vi "PIDAutoTune_ClosedLoopStep.vi"(7 "Configuration Parameters":T2={"Controller Constant Type"=enum."Ziegler Nicols - Normal", "Type of Controller"=enum."PI", "CO Offset"=0.25, "Kn"=1.0, "Tuning Tolerance"=0.001, "Plant Tolerance"=0.001, "Newest Avg Time "=1, "Long Ave Time"=6}, 8 "Sampling Time dt (s)":dbl=0.02, 9 "Tune":bool, 10 "Measurement  (PV)":dbl, 11 "Control Output (Co)":dbl) -> (0 "Plant and Test Data":T4, 1 "New Tuning Parameters":T3, 2 "Tuning Done":bool, 3 "Adj CO":dbl, 4 "Error Occured":bool, 6 "Diagnostic":T1)   [LabVIEW 2019, in "Trajectory_Library.lvlib"]
uses:
  Trajectory_Library.lvlib
  <vilib>/addons/control/pid/NI_PID_autopid.lvlib
  <vilib>/ptbypt/NI_PtbyPt.lvlib
  <vilib>/Analysis/Matrix/NI_Matrix.lvlib
  <vilib>/addons/control/pid/autopid.llb/PID Autotuning Design (Auto).vi
  <vilib>/addons/control/pid/autopid.llb/PID Autotuning Design (Chien-Hrones-Reswick).vi
  <vilib>/Analysis/Matrix/Numeric/Conversions/Array To Matrix - RA.vi
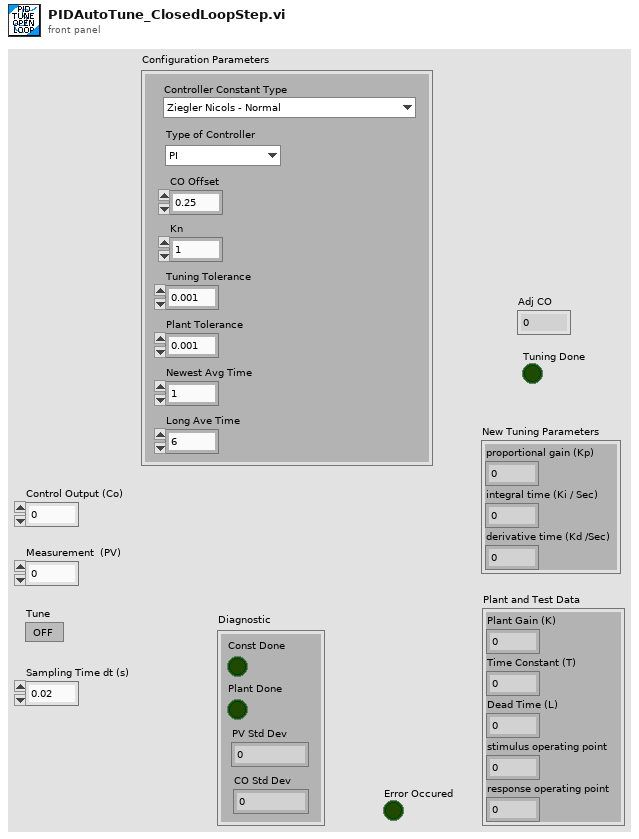
[diagram p1: front panel]
types:
  T1 = cluster{"Const Done":bool, "Plant Done":bool, "PV Std Dev":dbl, "CO Std Dev":dbl}
  T2 = cluster{"Controller Constant Type":enum16{"Ziegler Nicols - Fast", "Ziegler Nicols - Normal", "Ziegler Nicols - Slow", "CHR regulator - 0% overshoot", "CHR regulator - 20% overshoot", "CHR servo - 0 % overshoot", "CHR servo - 20% overshoot"}, "Type of Controller":enum16{"P", "PI", "PID"}, "CO Offset":dbl, "Kn":dbl, "Tuning Tolerance":dbl, "Plant Tolerance":dbl, "Newest Avg Time ":i32, "Long Ave Time":i32}
  T3 = cluster{"proportional gain (Kp)":dbl, "integral time (Ki / Sec)":dbl, "derivative time (Kd /Sec)":dbl}
  T4 = cluster{"Plant Gain (K)":dbl, "Time Constant (T)":dbl, "Dead Time (L)":dbl, "stimulus operating point":dbl, "response operating point":dbl}
  T5 = enum16{"Moving Average", "Low Pass 1st Order Butterworth", "Low Pass 2nd Order Butterworth", "High Pass 1st Order Butterworth", "High Pass 2nd Order Butterworth"}
  T6 = enum16{"Ziegler Nicols - Fast", "Ziegler Nicols - Normal", "Ziegler Nicols - Slow", "CHR regulator - 0% overshoot", "CHR regulator - 20% overshoot", "CHR servo - 0 % overshoot", "CHR servo - 20% overshoot"}
  T7 = cluster{"proportional gain (Kc)":dbl, "integral time (Ti, min)":dbl, "derivative time (Td, min)":dbl}
  T8 = cluster{"Plant Gain (K)":dbl, "Time Constant (T)":dbl, "Dead Time (L)":dbl}
  T9 = cluster{"Plant Gain (K)":dbl, "Time Constant (T)":dbl, "Dead Time (L)":dbl, "stimulus offset":dbl, "response offset":dbl}
  T10 = typedef "NI_Matrix.lvlib/RealMatrix.ctl" = dbl[][]
  T11 = cluster{"WithinTolerance":bool, "WithinTolerance":bool, "standard deviation":dbl, "standard deviation":dbl}
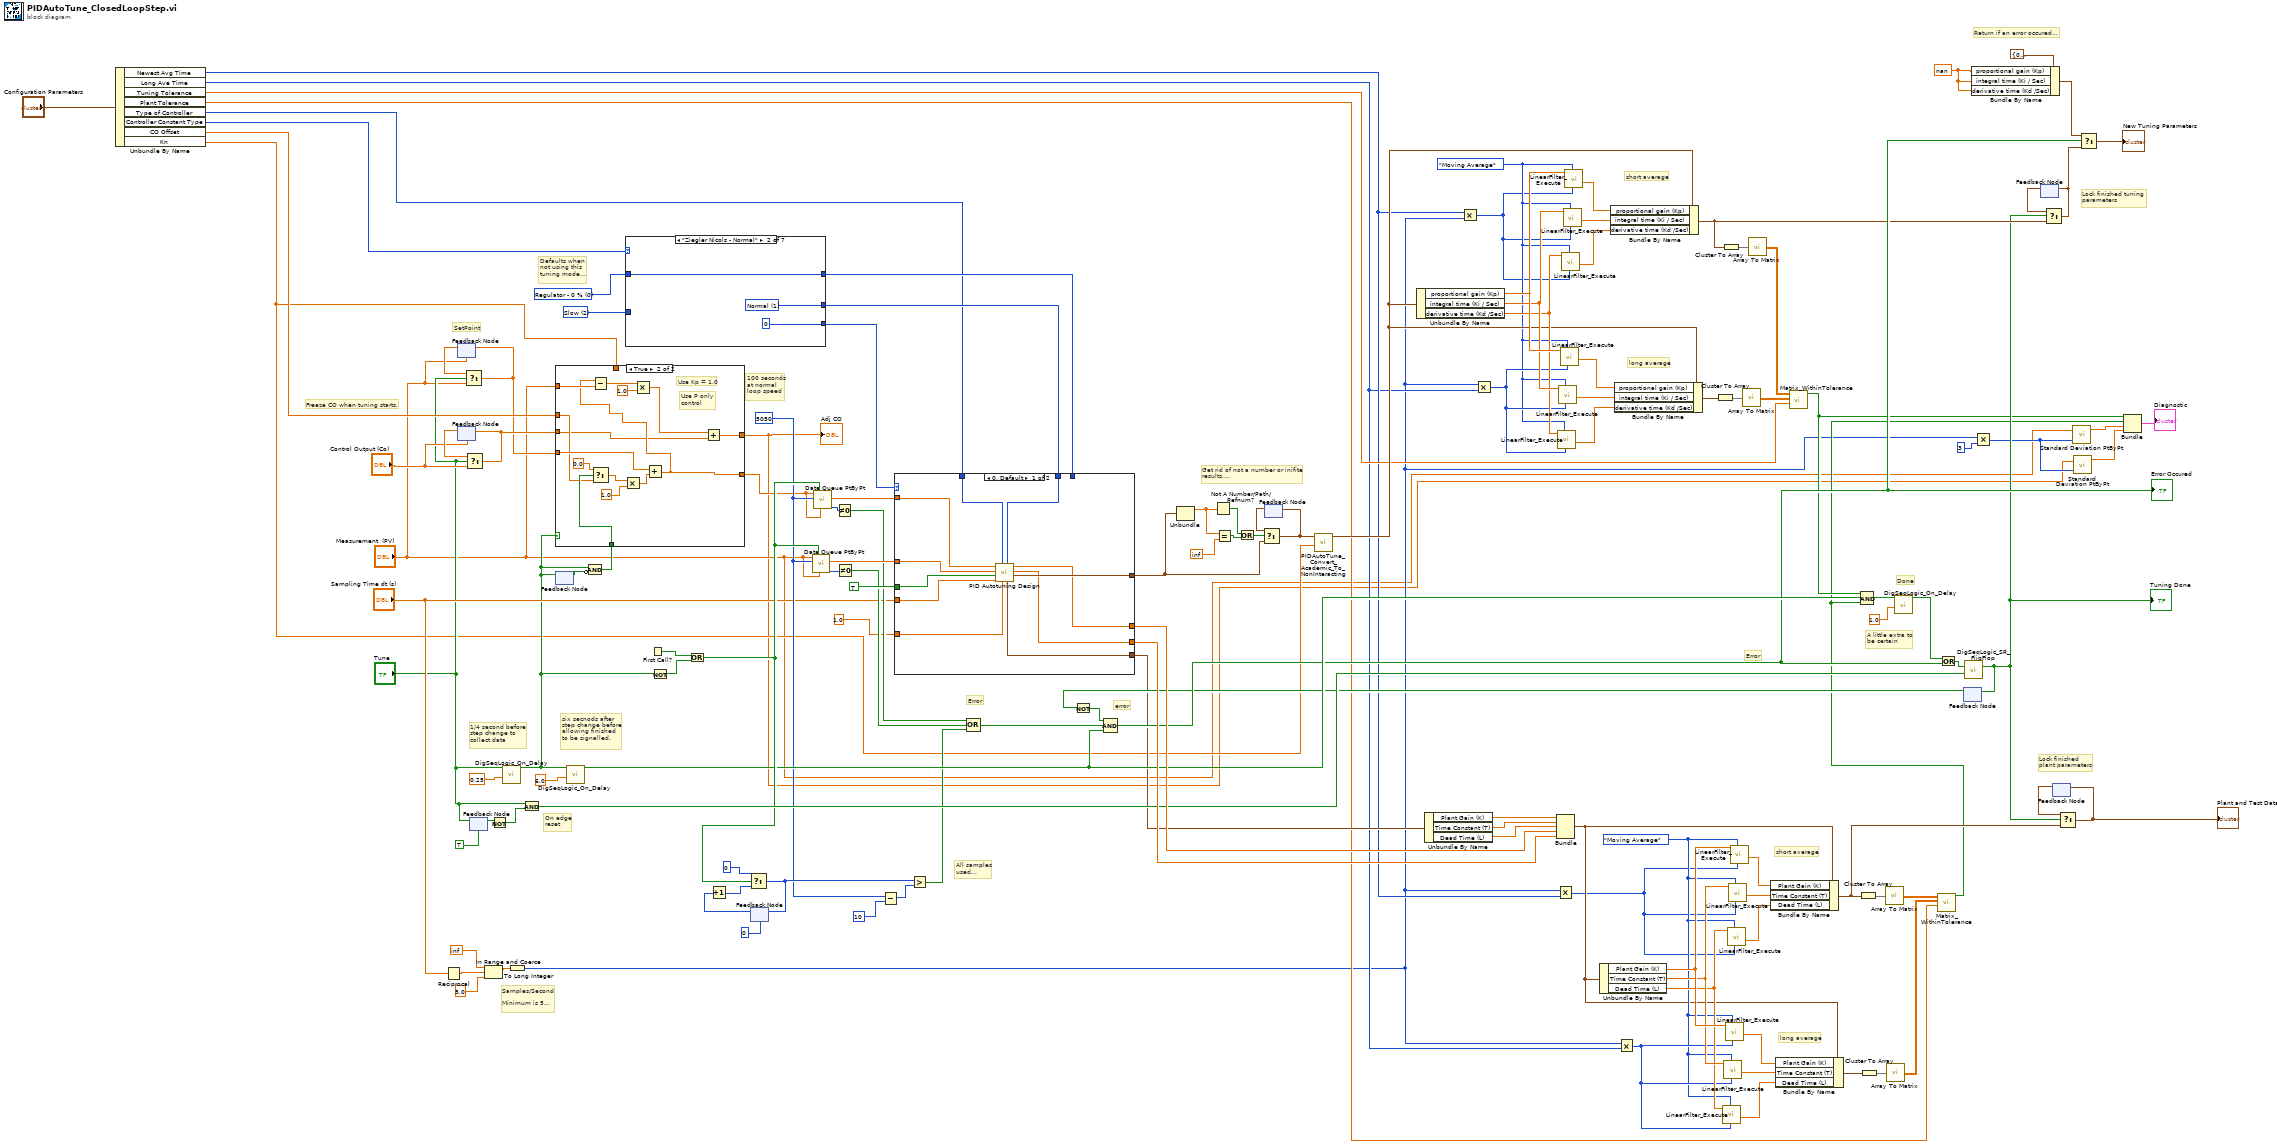
[diagram p0: block diagram]
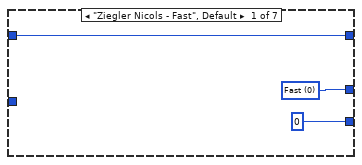
[diagram p2: hidden frame]
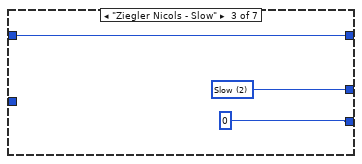
[diagram p3: hidden frame]
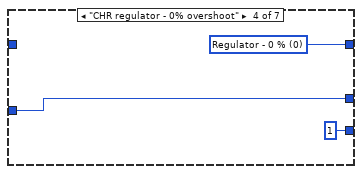
[diagram p4: hidden frame]
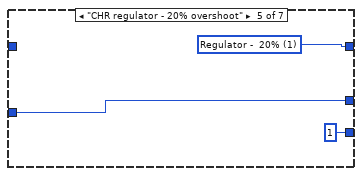
[diagram p5: hidden frame]
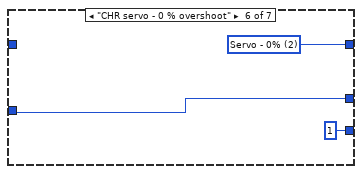
[diagram p6: hidden frame]
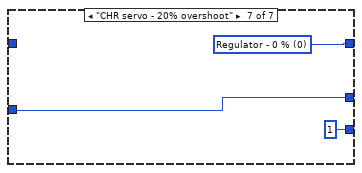
[diagram p7: hidden frame]
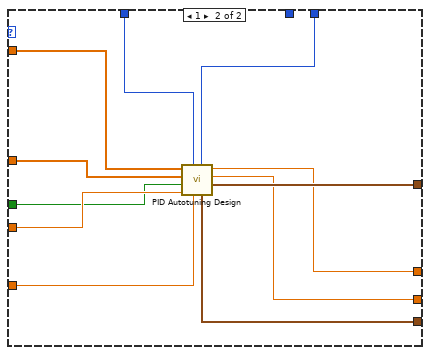
[diagram p8: hidden frame]
diagram:
  w39 = T5."Moving Average" ("Filter Type")
  w91 = nan
  w50 = T5."Moving Average" ("Filter Type")
  w106 = u16 2 items=["Fast", "Normal", "Slow"] ("Ziegler-Nichols Speed")
  w107 = u16 0 items=["Regulator - 0 %", "Regulator -  20%", "Servo - 0%", "Servo - 20%"] ("Tuning specifications")
  w78 = 5050 ("sample length")
  # "SetPoint"
  # "Get rid of not a number or inifite\nresults...."
  # "On edge\nreset"
  # "Error"
  # "All samples\nused..."
  # "Error"
  # "Done"
  # "Lock finished \nplant parameters"
  # "Lock finished tuning\nparameters"
  # "Samples/Second\n\nMinimum is 5..."
  # "long average"
  # "short average"
  # "long average"
  # "short average"
  # "error"
  # "Return if an error occured..."
  # "A little extra to\nbe certain"
  # "Defaults when\nnot using this\ntuning mode..."
  # "100 seconds\nat normal\nloop speed"
  # "Freeze CO when tuning starts."
  # "six secnods after\nstep change before\nallowing finished \nto be signalled."
  # "1/4 second before\nstep change to\ncollect data"
  n1 = Unbundle By Name("Configuration Parameters") -> ("Newest Avg Time"=w21:i32, "Long Ave Time"=w20:i32, "Tuning Tolerance"=w26:dbl, "Plant Tolerance"=w25:dbl, "Type of Controller"=w28:enum16{"P", "PI", "PID"}, "Controller Constant Type"=w29:T6, "CO Offset"=w27:dbl, "Kn"=w9:dbl)
  n2 = Reciprocal(x="Sampling Time dt (s)") -> (1/x=w68:dbl)
  n3 = feedback #1("Measurement  (PV)") -> (w16:dbl)
  n4 = feedback #2("Control Output (Co)") -> (w121:dbl)
  n5 = Select(t=w16, s="Tune", f="Measurement  (PV)") -> (s? t:f=w14:dbl)
  n6 = feedback-in #1(w14) -> ()
  n7 = Select(t=w121, s="Tune", f="Control Output (Co)") -> (s? t:f=w122:dbl)
  n8 = feedback-in #2(w122) -> ()
  n9 = feedback-in #3("Tune") -> ()
  n10 = feedback #3(TRUE ("Tune")) -> (w118:bool)
  n11 = In Range and Coerce(upper limit=inf, x=w68, lower limit=5.0) -> (coerced(x)=w59:dbl)  [unwired: 1 out]
  n12 = Not(x=w118) -> (.not. x?=w117:bool)
  n13 = call "DigSeqLogic_On_Delay.vi"("Delay"=0.25, "Input"="Tune") -> ("Output"=w10:bool)  [unwired: 8 in, 1 out]
  n14 = To Long Integer(number=w59) -> (32bit integer=w5:i32)
  n15 = And(x="Tune", y=w117) -> (x .and. y?=w116:bool)
  n16 = feedback-in #4(w10) -> ()
  n17 = feedback #4() -> (w13:bool)  [unwired: 1 in]
  n18 = call "DigSeqLogic_On_Delay.vi"("Delay"=6.0, "Input"=w10) -> ("Output"=w85:bool)  [unwired: 8 in, 1 out]
  n19 = Compound Arithmetic op=AND(w10, invert w13) -> (w12:bool)
  n20 = case shown="True" w10 {
    tunnel: w122 -> [w137 w142]
    tunnel: w27 -> [_ w143]
    tunnel: [w137 w148] -> w1
    tunnel: w14 -> [w136 w145]
    tunnel: "Measurement  (PV)" -> [_ w151]
    tunnel: w12 -> [_ w146]
    tunnel: [w136 w144] -> w11
    tunnel: w9 -> [_ _]
    frame False {
    }
    frame True {
      # "Use P only \ncontrol"
      # "Use Kp = 1.0"
      n21 = Select(t=0.0, s=w146, f=w143) -> (s? t:f=w139:dbl)
      n22 = Multiply(x=w139, y=1.0) -> (x*y=w141:dbl)
      n23 = Add(x=w145, y=w141) -> (x+y=w144:dbl)
      n24 = Subtract(x=w144, y=w151) -> (x-y=w150:dbl)
      n25 = Multiply(x=w150, y=1.0) -> (x*y=w149:dbl)
      n26 = Add(x=w149, y=w142) -> (x+y=w148:dbl)
    }
  }
  "Adj CO" <- w1
  n27 = case shown="\"Ziegler Nicols - Normal\"" w29 {
    tunnel: [w154 w157 w160 w161 w164 w167 w170] -> w110
    tunnel: [0 0 0 1 1 1 1] -> w109
    tunnel: [w152 w155 w158 w162 w165 w168 w171] -> w108
    tunnel: w107 -> [w152 w155 w158 _ _ _ _]
    tunnel: w106 -> [_ _ _ w161 w164 w167 w170]
    frame "Ziegler Nicols - Fast", Default {
      w154 = u16 0 items=["Fast", "Normal", "Slow"] ("Ziegler-Nichols Speed")
    }
    frame "Ziegler Nicols - Normal" {
      w157 = u16 1 items=["Fast", "Normal", "Slow"] ("Ziegler-Nichols Speed")
    }
    frame "Ziegler Nicols - Slow" {
      w160 = u16 2 items=["Fast", "Normal", "Slow"] ("Ziegler-Nichols Speed")
    }
    frame "CHR regulator - 0% overshoot" {
      w162 = u16 0 items=["Regulator - 0 %", "Regulator -  20%", "Servo - 0%", "Servo - 20%"] ("Tuning specifications")
    }
    frame "CHR regulator - 20% overshoot" {
      w165 = u16 1 items=["Regulator - 0 %", "Regulator -  20%", "Servo - 0%", "Servo - 20%"] ("Tuning specifications")
    }
    frame "CHR servo - 0 % overshoot" {
      w168 = u16 2 items=["Regulator - 0 %", "Regulator -  20%", "Servo - 0%", "Servo - 20%"] ("Tuning specifications")
    }
    frame "CHR servo - 20% overshoot" {
      w171 = u16 0 items=["Regulator - 0 %", "Regulator -  20%", "Servo - 0%", "Servo - 20%"] ("Tuning specifications")
    }
  }
  n28 = First Call?() -> (First Call?: T/F=w90:bool)
  n29 = Not(x=w10) -> (.not. x?=w89:bool)
  n30 = Or(x=w90, y=w89) -> (x .or. y?=w87:bool)
  n31 = feedback #5(0) -> (w82:i32)
  n32 = Increment(x=w82) -> (x+1=w81:i32)
  n33 = Select(t=0, s=w87, f=w81) -> (s? t:f=w80:i32)
  n34 = feedback-in #5(w80) -> ()
  n35 = call <vilib>:"Data Queue PtByPt.vi"("initial queue element"="Measurement  (PV)", "initialize"=w87, "sample length"=w78, "input data point"="Measurement  (PV)") -> ("error"=w98:i32, "Current Queue"=w130:dbl[])  [unwired: 3 in, 3 out]
  n36 = call <vilib>:"Data Queue PtByPt.vi"("initial queue element"=w11, "initialize"=w87, "sample length"=w78, "input data point"=w11) -> ("error"=w99:i32, "Current Queue"=w131:dbl[])  [unwired: 3 in, 3 out]
  n37 = Not Equal To 0?(x=w99) -> (x != 0?=w75:bool)
  n38 = Not Equal To 0?(x=w98) -> (x != 0?=w74:bool)
  n39 = Subtract(x=w78, y=10) -> (x-y=w79:i32)
  n40 = case shown="0, Default" w109 {
    tunnel: [w183 w194] -> w134
    tunnel: "Sampling Time dt (s)" -> [w182 w193]
    tunnel: w131 -> [w181 w192]
    tunnel: w130 -> [w180 w191]
    tunnel: w28 -> [w179 w190]
    tunnel: [w173 w189] -> w38
    tunnel: [w178 w188] -> w126
    tunnel: [w177 w187] -> w125
    tunnel: 1.0 ("Kn") -> [w176 w186]
    tunnel: w110 -> [w175 _]
    tunnel: w108 -> [_ w185]
    tunnel: TRUE ("closed-loop?") -> [w174 w184]
    frame 0, Default {
      n41 = call-poly <vilib>:"PID Autotuning Design.vi"("Ziegler-Nichols Speed"=w175, "Controller Gain (K)"=w176, "Type of Controller"=w179, "dt (s)"=w182, "closed-loop?"=w174, "Response signal"=w180, "Stimulus signal"=w181) -> ("PID gains"=w183:T7, "response operating point"=w177:dbl, "stimulus operating point"=w178:dbl, "Plant Parameters"=w173:T8)  [unwired: 1 in]
    }
    frame 1 {
      n42 = call-poly <vilib>:"PID Autotuning Design.vi"("Tuning specifications"=w185, "Controller Gain (K)"=w186, "Type of Controller"=w190, "dt (s)"=w193, "closed-loop?"=w184, "Response signal"=w191, "Stimulus signal"=w192) -> ("PID gains"=w194:T7, "response offset"=w187:dbl, "stimulus offset"=w188:dbl, "Plant Parameters"=w189:T8)  [unwired: 1 in]
    }
  }
  n43 = Greater?(x=w80, y=w79) -> (0:w76:bool)
  n44 = Compound Arithmetic op=OR(w75, w74, w76) -> (w86:bool)
  n45 = Unbundle(w134) -> ("proportional gain (Kc)"=w71:dbl)  [unwired: 2 out]
  n46 = Not A Number/Path/Refnum?(number/path/refnum=w71) -> (NaN/Path/Refnum?=w70:bool)
  n47 = Equal?(x=w71, y=inf) -> (x = y?=w100:bool)
  n48 = Or(x=w70, y=w100) -> (x .or. y?=w101:bool)
  n49 = feedback #6() -> (w133:T7)  [unwired: 1 in]
  n50 = Select(t=w133, s=w101, f=w134) -> (s? t:f=w135:T7)
  n51 = feedback-in #6(w135) -> ()
  n52 = call "PIDAutoTune_Convert_Academic_To_NonInteracting.vi"("Kn"=w9, "PID gains NI Academic"=w135) -> ("PID Gains Non Interacting"=w55:T3)  [unwired: 9 in]
  n53 = Unbundle By Name(w55) -> ("proportional gain (Kp)"=w62:dbl, "integral time (Ki / Sec)"=w61:dbl, "derivative time (Kd /Sec)"=w60:dbl)
  n54 = Unbundle By Name(w38) -> ("Plant Gain (K)"=w129:dbl, "Time Constant (T)"=w128:dbl, "Dead Time (L)"=w127:dbl)
  n55 = Multiply(x=w21, y=w5) -> (x*y=w24:i32)
  n56 = Multiply(x=w5, y=w20) -> (x*y=w58:i32)
  n57 = Bundle("Plant Gain (K)"=w129, "Time Constant (T)"=w128, "Dead Time (L)"=w127, "stimulus offset"=w126, "response offset"=w125) -> (w37:T9)  [unwired: 1 in]
  n58 = Multiply(x=w5, y=w21) -> (x*y=w22:i32)
  n59 = call "LinearFilter_Execute.vi"("Samples"=w58, "Filter Type"=w50, "Input"=w60) -> ("Output"=w63:dbl)  [unwired: 7 in, 1 out]
  n60 = call "LinearFilter_Execute.vi"("Samples"=w58, "Filter Type"=w50, "Input"=w61) -> ("Output"=w65:dbl)  [unwired: 7 in, 1 out]
  n61 = call "LinearFilter_Execute.vi"("Samples"=w58, "Filter Type"=w50, "Input"=w62) -> ("Output"=w64:dbl)  [unwired: 7 in, 1 out]
  n62 = call "LinearFilter_Execute.vi"("Samples"=w24, "Filter Type"=w50, "Input"=w60) -> ("Output"=w102:dbl)  [unwired: 7 in, 1 out]
  n63 = call "LinearFilter_Execute.vi"("Samples"=w24, "Filter Type"=w50, "Input"=w61) -> ("Output"=w103:dbl)  [unwired: 7 in, 1 out]
  n64 = call "LinearFilter_Execute.vi"("Samples"=w24, "Filter Type"=w50, "Input"=w62) -> ("Output"=w104:dbl)  [unwired: 7 in, 1 out]
  n65 = Unbundle By Name(w37) -> ("Plant Gain (K)"=w43:dbl, "Time Constant (T)"=w42:dbl, "Dead Time (L)"=w41:dbl)
  n66 = Bundle By Name(cluster=w55, "proportional gain (Kp)"=w104, "integral time (Ki / Sec)"=w103, "derivative time (Kd /Sec)"=w102) -> (w54:T3)
  n67 = Bundle By Name(cluster=w55, "proportional gain (Kp)"=w64, "integral time (Ki / Sec)"=w65, "derivative time (Kd /Sec)"=w63) -> (w57:T3)
  n68 = Multiply(x=w5, y=w20) -> (x*y=w40:i32)
  n69 = Cluster To Array(cluster=w57) -> (array=w56:dbl[])
  n70 = Cluster To Array(cluster=w54) -> (array=w53:dbl[])
  n71 = call "LinearFilter_Execute.vi"("Samples"=w40, "Filter Type"=w39, "Input"=w41) -> ("Output"=w44:dbl)  [unwired: 7 in, 1 out]
  n72 = call "LinearFilter_Execute.vi"("Samples"=w40, "Filter Type"=w39, "Input"=w42) -> ("Output"=w46:dbl)  [unwired: 7 in, 1 out]
  n73 = call "LinearFilter_Execute.vi"("Samples"=w40, "Filter Type"=w39, "Input"=w43) -> ("Output"=w45:dbl)  [unwired: 7 in, 1 out]
  n74 = call "LinearFilter_Execute.vi"("Samples"=w22, "Filter Type"=w39, "Input"=w41) -> ("Output"=w47:dbl)  [unwired: 7 in, 1 out]
  n75 = call "LinearFilter_Execute.vi"("Samples"=w22, "Filter Type"=w39, "Input"=w42) -> ("Output"=w48:dbl)  [unwired: 7 in, 1 out]
  n76 = call "LinearFilter_Execute.vi"("Samples"=w22, "Filter Type"=w39, "Input"=w43) -> ("Output"=w49:dbl)  [unwired: 7 in, 1 out]
  n77 = call-poly <vilib>:"Array To Matrix.vi"("Real 1D Array"=w56) -> ("Real Matrix (Column Vector)"=w52:T10)
  n78 = call-poly <vilib>:"Array To Matrix.vi"("Real 1D Array"=w53) -> ("Real Matrix (Column Vector)"=w51:T10)
  n79 = Bundle By Name(cluster=w37, "Plant Gain (K)"=w49, "Time Constant (T)"=w48, "Dead Time (L)"=w47) -> (w33:T9)
  n80 = Bundle By Name(cluster=w37, "Plant Gain (K)"=w45, "Time Constant (T)"=w46, "Dead Time (L)"=w44) -> (w34:T9)
  n81 = call "Matrix_WithinTolerance.vi"("Tolerance"=w26, "Matrix B"=w52, "Matrix A"=w51) -> ("WithinTolerance"=w18:bool)  [unwired: 7 in, 1 out]
  n82 = Cluster To Array(cluster=w33) -> (array=w36:dbl[])
  n83 = Cluster To Array(cluster=w34) -> (array=w35:dbl[])
  n84 = call-poly <vilib>:"Array To Matrix.vi"("Real 1D Array"=w36) -> ("Real Matrix (Column Vector)"=w32:T10)
  n85 = call-poly <vilib>:"Array To Matrix.vi"("Real 1D Array"=w35) -> ("Real Matrix (Column Vector)"=w31:T10)
  n86 = call "Matrix_WithinTolerance.vi"("Tolerance"=w25, "Matrix B"=w31, "Matrix A"=w32) -> ("WithinTolerance"=w17:bool)  [unwired: 7 in, 1 out]
  n87 = Compound Arithmetic op=AND(w18, w85, w17) -> (w112:bool)
  n88 = call "DigSeqLogic_On_Delay.vi"("Delay"=1.0, "Input"=w112) -> ("Output"=w96:bool)  [unwired: 8 in, 1 out]
  n89 = feedback #7() -> (w72:bool)  [unwired: 1 in]
  n90 = Not(x=w72) -> (.not. x?=w73:bool)
  n91 = Compound Arithmetic op=AND(w73, w86, w85) -> (w84:bool)
  "Error Occured" <- w84
  n92 = Or(x=w96, y=w84) -> (x .or. y?=w97:bool)
  n93 = call "DigSeqLogic_SR_FlipFlop.vi"("Set"=w97, "Reset"=w116) -> ("Output"=w23:bool)  [unwired: 12 in, 1 out]
  "Tuning Done" <- w23
  n94 = feedback-in #7(w23) -> ()
  n95 = Bundle By Name(cluster=T3 {"proportional gain (Kp)"=0.0, "integral time (Ki / Sec)"=0.0, "derivative time (Kd /Sec)"=0.0} ("t"), "proportional gain (Kp)"=w91, "integral time (Ki / Sec)"=w91, "derivative time (Kd /Sec)"=w91) -> (w92:T3)
  n96 = Multiply(x=w5, y=3) -> (x*y=w6:i32)
  n97 = feedback #8() -> (w113:T3)  [unwired: 1 in]
  n98 = Select(t=w113, s=w23, f=w54) -> (s? t:f=w94:T3)
  n99 = feedback-in #8(w94) -> ()
  n100 = feedback #9() -> (w114:T9)  [unwired: 1 in]
  n101 = Select(t=w114, s=w23, f=w33) -> (s? t:f=w115:T9)
  "Plant and Test Data" <- w115
  n102 = feedback-in #9(w115) -> ()
  n103 = call <vilib>:"Standard Deviation PtByPt.vi"("x"="Measurement  (PV)", "sample length"=w6) -> ("standard deviation"=w4:dbl)  [unwired: 1 in, 2 out]
  n104 = call <vilib>:"Standard Deviation PtByPt.vi"("x"=w1, "sample length"=w6) -> ("standard deviation"=w3:dbl)  [unwired: 1 in, 2 out]
  n105 = Select(t=w92, s=w84, f=w94) -> (s? t:f=→"New Tuning Parameters":T3)
  n106 = Bundle("WithinTolerance"=w18, "WithinTolerance"=w17, "standard deviation"=w4, "standard deviation"=w3) -> (→"Diagnostic":T11)  [unwired: 1 in]
